vi "DataTreeCtrlFM writeData.vi"(7 "sampleType":string="Untitled", 8 "error IO":errorcluster, 10 "SignalData":waveform(sgl), 11 "TDMSAdv Class in":refnum<class "TDMSAdv.lvclass">) -> (0 "error out":errorcluster, 3 "TDMSAdv Class out":refnum<class "TDMSAdv.lvclass">)   [LabVIEW 2018, in "DataTreeCtrl.lvclass"]
uses:
  DataTreeCtrl.lvclass
  PublicSubVI/Class/FileManager/TDMSAdv.lvclass
  PublicSubVI/Class/FileManager/TDMSAdv/TDMSAdv writeOfString.vi
  PublicSubVI/Class/FileManager/TDMSAdv/TDMSAdv writeOfDBL.vi
  PublicSubVI/Class/FileManager/TDMSAdv/TDMSAdv writeOfSGL.vi
  PublicSubVI/Class/FileManager/FM.lvclass
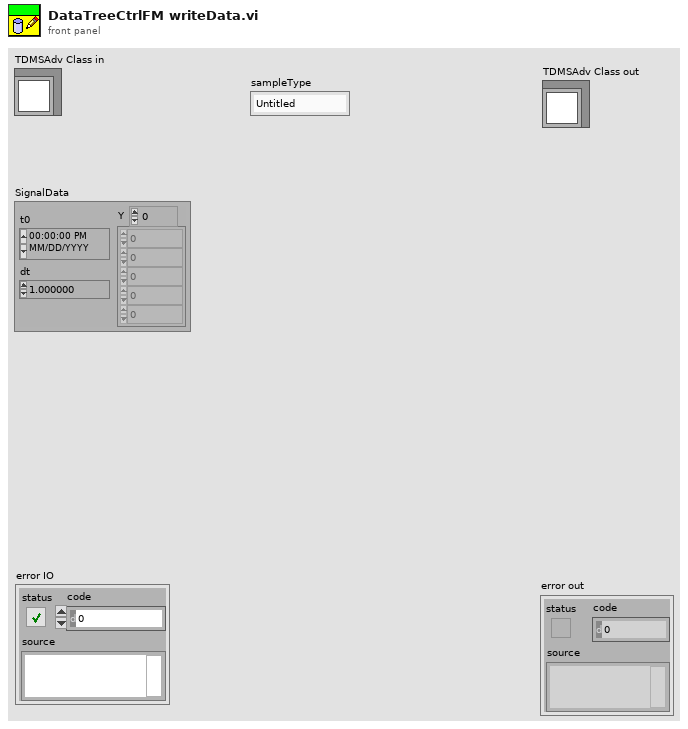
[diagram p1: front panel]
types:
  T1 = cluster{"attrData":string, "mzRange":string, "dt":dbl, "yData":sgl[], "dataTime":timestamp}
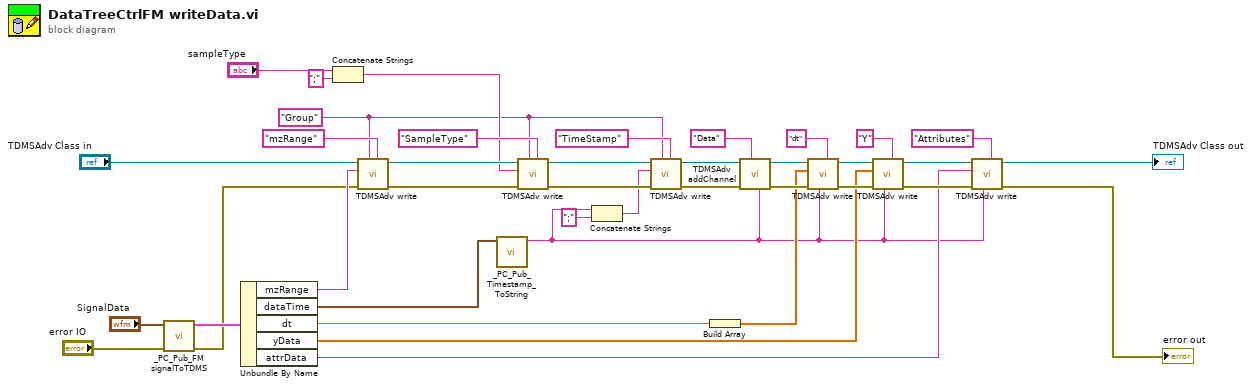
[diagram p0: block diagram]
diagram:
  w2 = "Group" ("group name (Untitled)")
  n1 = call "_PC_Pub_FM signalToTDMS.vi"("error in (no error)"="error IO", "SignalData"="SignalData") -> ("error out"=w1:errorcluster, "dataParam"=w6:T1)  [unwired: 7 in, 1 out]
  n2 = Unbundle By Name(w6) -> ("mzRange"=w3:string, "dataTime"=w13:timestamp, "dt"=w12:dbl, "yData"=w11:sgl[], "attrData"=w10:string)
  n3 = Concatenate Strings("sampleType", ";" ("string")) -> (w17:string)
  n4 = call-poly "TDMSAdv write.vi"("channel name"="mzRange", "group name (Untitled)"=w2, "error in (no error)"=w1, "dataArray"=w3, "TDMSAdv in"="TDMSAdv Class in") -> ("error out"=w30:errorcluster, "TDMSAdv out"=w31:refnum<class "TDMSAdv.lvclass">)  [unwired: 5 in]
  n5 = call "_PC_Pub_Timestamp_ToString.vi"("Timestamp"=w13) -> ("Timestring"=w8:string)  [unwired: 9 in, 1 out]
  n6 = call-poly "TDMSAdv write.vi"("channel name"="SampleType", "group name (Untitled)"=w2, "error in (no error)"=w30, "dataArray"=w17, "TDMSAdv in"=w31) -> ("error out"=w34:errorcluster, "TDMSAdv out"=w33:refnum<class "TDMSAdv.lvclass">)  [unwired: 5 in]
  n7 = Concatenate Strings(w8, ";" ("string")) -> (w14:string)
  n8 = call-poly "TDMSAdv write.vi"("channel name"="TimeStamp", "group name (Untitled)"=w2, "error in (no error)"=w34, "dataArray"=w14, "TDMSAdv in"=w33) -> ("error out"=w21:errorcluster, "TDMSAdv out"=w22:refnum<class "TDMSAdv.lvclass">)  [unwired: 5 in]
  n9 = Build Array(w12) -> (w16:dbl[])
  n10 = call "TDMSAdv addChannel.vi"("channel name"=w8, "group name (Untitled)"="Data" ("channel name"), "error in (no error)"=w21, "TDMSAdv in"=w22) -> ("error out"=w19:errorcluster, "TDMSAdv out"=w20:refnum<class "TDMSAdv.lvclass">)  [unwired: 6 in]
  n11 = call-poly "TDMSAdv write.vi"("channel name"="dt", "group name (Untitled)"=w8, "error in (no error)"=w19, "dataArray"=w16, "TDMSAdv in"=w20) -> ("error out"=w24:errorcluster, "TDMSAdv out"=w25:refnum<class "TDMSAdv.lvclass">)  [unwired: 5 in]
  n12 = call-poly "TDMSAdv write.vi"("channel name"="Y", "group name (Untitled)"=w8, "error in (no error)"=w24, "dataArray"=w11, "TDMSAdv in"=w25) -> ("error out"=w28:errorcluster, "TDMSAdv out"=w27:refnum<class "TDMSAdv.lvclass">)  [unwired: 5 in]
  n13 = call-poly "TDMSAdv write.vi"("channel name"="Attributes", "group name (Untitled)"=w8, "error in (no error)"=w28, "dataArray"=w10, "TDMSAdv in"=w27) -> ("error out"=→"error out":errorcluster, "TDMSAdv out"=→"TDMSAdv Class out":refnum<class "TDMSAdv.lvclass">)  [unwired: 5 in]
